vi "InitDone.vi"(8 "error in (no error)":errorcluster, 9 "instr error":errorcluster, 10 "Address":T2, 11 "InterferometryUI in":refnum<class "InterferometryUI.lvclass">) -> (0 "error out":errorcluster, 3 "InterferometryUI out":refnum<class "InterferometryUI.lvclass">)   [LabVIEW 2023, in "InterferometryUI.lvlib" / "InterferometryUI.lvclass"]
uses:
  InterferometryUI.lvclass
  instrumentType.ctl
  InterferometryUI.lvclass/InterferometryUI.ctl
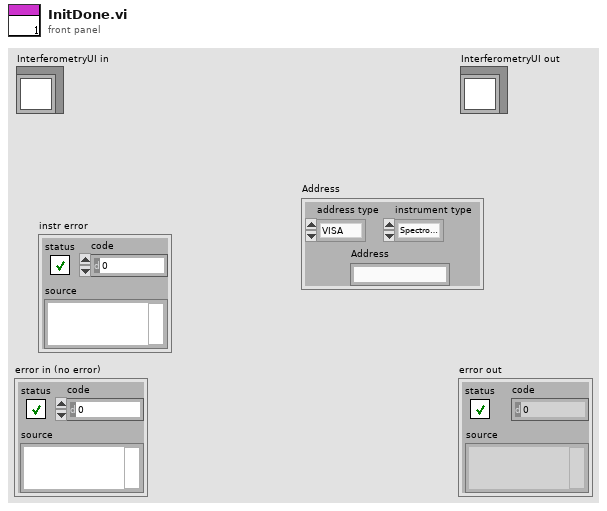
[diagram p1: front panel]
types:
  T1 = typedef "instrumentType.ctl" = enum16{"Spectrometer", "Camera", "Stepper"}
  T2 = cluster{"address type":enum16{"VISA", "Index"}, "Address":string, "instrument type":T1}
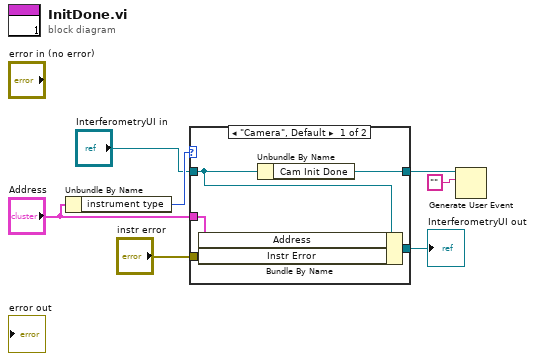
[diagram p0: block diagram]
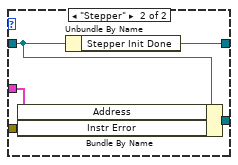
[diagram p2: hidden frame]
diagram:
  n1 = Unbundle By Name("Address") -> ("instrument type"=w6:T1)
  n2 = case shown="\"Camera\", Default" w6 {
    tunnel: "InterferometryUI in" -> [w11 w14]
    tunnel: [w12 w17] -> w4
    tunnel: [w10 w13] -> w3
    tunnel: "Address" -> [w8 w16]
    tunnel: "instr error" -> [w9 w15]
    frame "Camera", Default {
      n3 = Bundle By Name(cluster=w11, "Address"=w8, "Instr Error"=w9) -> (w10:refnum<class "InterferometryUI.lvclass">)
      n4 = Unbundle By Name(w11) -> ("Cam Init Done"=w12:refnum<user-event>)
    }
    frame "Stepper" {
      n5 = Bundle By Name(cluster=w14, "Address"=w16, "Instr Error"=w15) -> (w13:refnum<class "InterferometryUI.lvclass">)
      n6 = Unbundle By Name(w14) -> ("Stepper Init Done"=w17:refnum<user-event>)
    }
  }
  "InterferometryUI out" <- w3
  n7 = Generate User Event(user event=w4, event data cluster="" ("event data")) -> ()  [unwired: 2 in, 2 out]
